vi "Write To String Delimiter.vi"(8 "error in (no error)":errorcluster, 10 "Delimiter":string, 11 "Abs_String 1D in":refnum<class "Abs_String 1D.lvclass">) -> (0 "error out":errorcluster, 3 "Abs_String 1D out":refnum<class "Abs_String 1D.lvclass">)   [LabVIEW 2019, in "Abs_String 1D.lvclass"]
uses:
  Abs_String 1D.lvclass
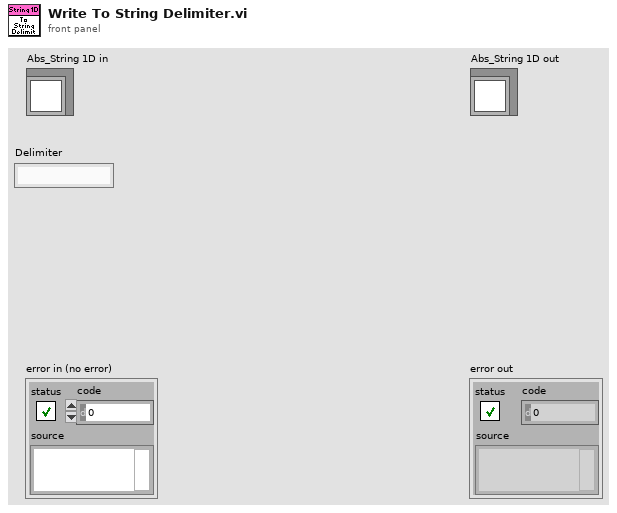
[diagram p1: front panel]
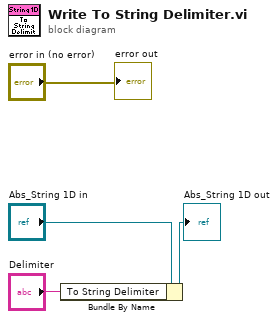
[diagram p0: block diagram]
diagram:
  n1 = Bundle By Name(cluster="Abs_String 1D in", "To String Delimiter"="Delimiter") -> (→"Abs_String 1D out":refnum<class "Abs_String 1D.lvclass">)
  "error out" <- "error in (no error)"
